vi "Uninstall Components.vi"(8 "Error In":errorcluster, 11 "Configuration in":T1) -> (0 "Error Out":errorcluster, 2 "Deleted Components":path[](array[path]), 3 "Configuration out":T1)   [LabVIEW 2011, in "LVH-Build-Tools.lvlib"]
uses:
  LVH-Build-Tools.lvlib
  Type Defs/Configuration.ctl
  Type Defs/Install Configuration.ctl
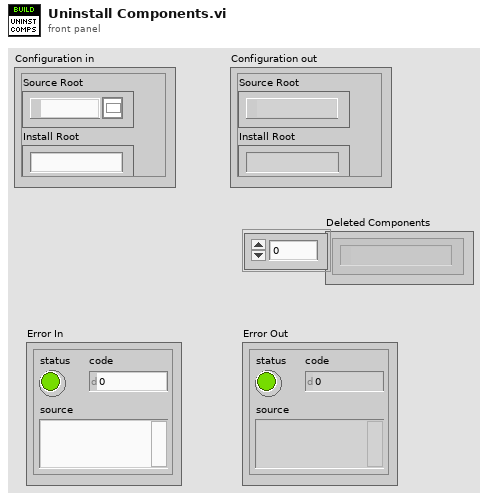
[diagram p1: front panel]
types:
  T1 = typedef "LVH-Build-Tools.lvlib/Configuration.ctl" = cluster{"Source Root":path, "Install Root":string, "Components":string[], "Ignore":string[], "Config Files":path[], "LV Directories":path[], "Install Paths":T2}
  T2 = typedef "LVH-Build-Tools.lvlib/Install Configuration.ctl" = cluster{"LabVIEW Directory":path, "Project Source Config":path}
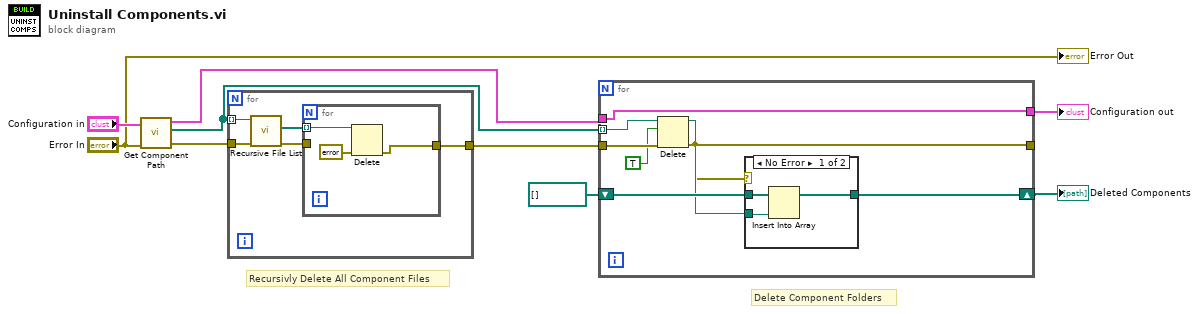
[diagram p0: block diagram]
diagram:
  # "Recursivly Delete All Component Files"
  # "Delete Component Folders"
  n1 = call "Get Component Path.vi"("Error In"="Error In", "Configuration"="Configuration in") -> ("Error Out"=w4:errorcluster, "Component Install Paths"=w2:path[], "Configuration"=w8:T1)  [unwired: 7 in]
  n2 = for {
    tunnel: w2 -> [w14] mode=indexing
    tunnel: w4 -> [w13]
    tunnel: [w10] -> w3
    n3 = call <vilib>:"Recursive File List.vi"("error in (no error)"=w13, "Folder Path"=w14) -> ("error out"=w11:errorcluster, "All Files in Dir"=w12:path[])  [unwired: 5 in, 3 out]
    n4 = for {
      tunnel: w12 -> [w17] mode=indexing
      tunnel: w11 -> [_]
      tunnel: [w16] -> w10
      n5 = Delete(path (use dialog)=w17, error in=errorcluster {"status"=FALSE, "code"=0, "source"=""}) -> (error out=w16:errorcluster)  [unwired: 3 in, 2 out]
    }
  }
  n6 = for {
    tunnel: w8 -> [w22]
    shift-right: [w20] -> w5
    shift-left: path[] [] -> [w25]
    tunnel: w2 -> [w18] mode=indexing
    tunnel: [w22] -> w6
    tunnel: w3 -> [w24]
    tunnel: [w19] -> _
    n7 = Delete(path (use dialog)=w18, entire hierarchy (F)=TRUE, error in=w24) -> (deleted path=w21:path, error out=w19:errorcluster)  [unwired: 2 in, 1 out]
    n8 = case shown="No Error" w19 {
      tunnel: w25 -> [w28 w29]
      tunnel: w21 -> [w27 _]
      tunnel: [w26 w29] -> w20
      frame No Error {
        n9 = Insert Into Array(array=w28, new element=w27) -> (w26:path[])  [unwired: 1 in]
      }
      frame Error {
      }
    }
  }
  "Configuration out" <- w6
  "Deleted Components" <- w5
  "Error Out" <- "Error In"
